vi "_073.vi"() -> ()   [LabVIEW 2024]
panel:
  out "indexing":i32[](array[numeric])
  out "i+1":i32
  out "o/p":i32
  out "o/p":i32
  out "i":i32
  # "Fundamentals :"
  # "2~>After running this VI,what is the value displayed in the o/p & iteration count?"
  # "Nrml Approach :"
  # "Dfrnt Approach :"
  # "( Work flow )"
  # "Check each number of the i/p array , if it is greater then 10 or Not ,if the number is not greater then 10 (the greater function return false & the val will sent to tunnel )& if the number is greater then 10 (the greater function return True , the loop will stop due to the condition terminal & returns the val that is greater then 10)\nif (MAX element is 5th position of the array The iteration count is 5 [why bcz normal iteration count is 4  and the increment fncn is connected to an iteration terminal ,so the o/p is 5"
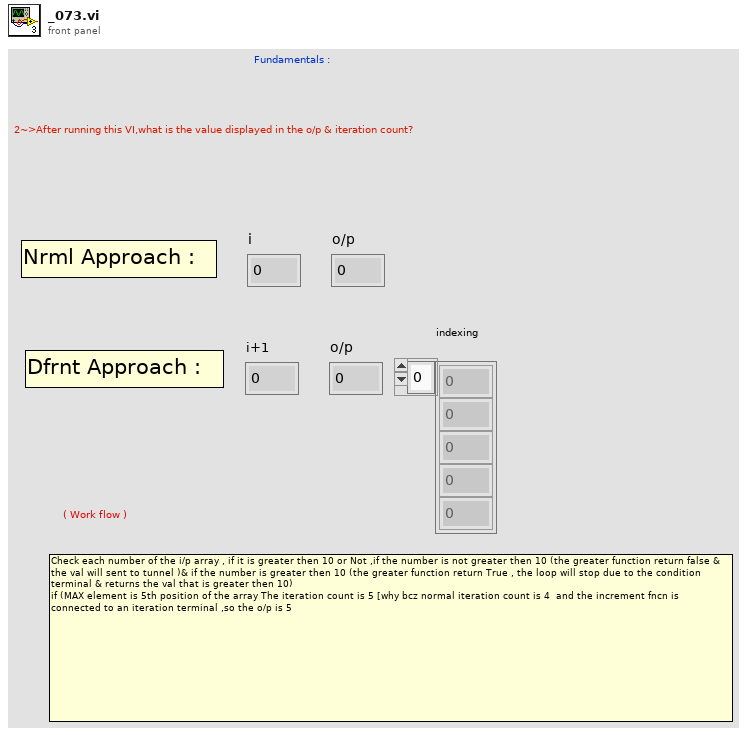
[diagram p1: front panel]
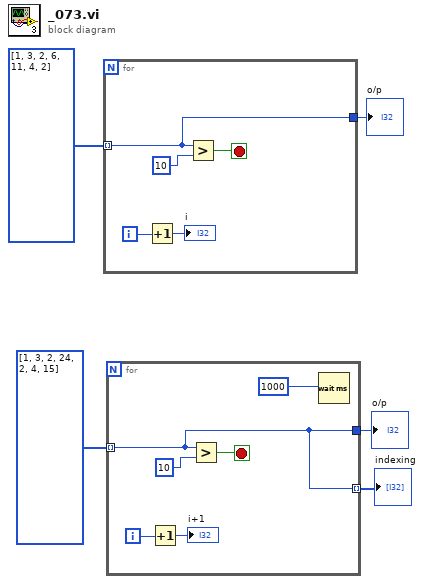
[diagram p0: block diagram]
diagram:
  n1 = for {
    tunnel: i32[] [1, 3, 2, 6, 11, 4, 2] -> [w6] mode=indexing
    tunnel: [w6] -> w4
    i -> [w9]
    stop <- w7 stop-if-true
    n2 = Increment(x=w9) -> (x+1=→"i":i32)
    n3 = Greater?(x=w6, y=10) -> (0:w7:bool)
  }
  "o/p" <- w4
  n4 = for {
    tunnel: i32[] [1, 3, 2, 24, 2, 4, 15] -> [w12] mode=indexing
    tunnel: [w12] -> w3
    tunnel: [w12] -> w1 mode=indexing
    i -> [w15]
    stop <- w13 stop-if-true
    n5 = Increment(x=w15) -> (x+1=→"i+1":i32)
    n6 = Greater?(x=w12, y=10) -> (0:w13:bool)
    n7 = Wait (ms)(milliseconds to wait=u32 1000 ("millisecond timer value")) -> ()  [unwired: 1 out]
  }
  "o/p" <- w3
  "indexing" <- w1
